vi "Write Send Functionality.vi"(6 "Message Priority":T1=enum."Normal", 7 "Publish Data?(T)":bool=TRUE, 8 "error in (no error)":errorcluster, 9 "Timeout if Waiting(-1ms)":i32=-1, 10 "Send Function(Await Reply)":T2=enum."Await Reply", 11 "Instrument Handler Reponse Msg in":refnum<class "Instrument Handler Response Msg.lvclass">) -> (0 "error out":errorcluster, 3 "Instrument Handler Reponse Msg out":refnum<class "Instrument Handler Response Msg.lvclass">)   [LabVIEW 2020, in "Instrument Handler.lvlib" / "Instrument Handler Response Msg.lvclass"]
doc: "Define the send functionality of the Instrument Handler Reponse Msg."
uses:
  Instrument Handler Response Msg.lvclass
  PPL/HDH.Actor Framework.Core.Publisher.lvlibp/Messages/Response Msg/Response Core/Controls/Ctl_SendFunction.ctl
  PPL/HDH.Actor Framework.Core.Actor.lvlibp/1abvi3w/vi.lib/ActorFramework/Message Enqueuer/Message Priority.ctl
  Instrument Handler Response Msg.lvclass/Instrument Handler Response Msg.ctl
  PPL/HDH.Actor Framework.Core.Publisher.lvlibp
  PPL/HDH.Actor Framework.Core.Actor.lvlibp/1abvi3w/vi.lib/ActorFramework/Message Enqueuer/Message Enqueuer.lvclass
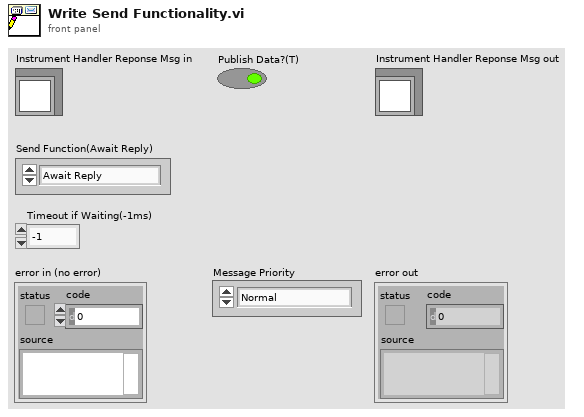
[diagram p1: front panel]
types:
  T1 = typedef "HDH.Actor Framework.Core.Actor.lvlibp/Message Enqueuer.lvclass/Message Priority.ctl" = enum16{"Low", "Normal", "High"}
  T2 = typedef "HDH.Actor Framework.Core.Publisher.lvlibp/Ctl_SendFunction.ctl" = enum16{"Send and Forget", "Request Reply", "Await Reply"}
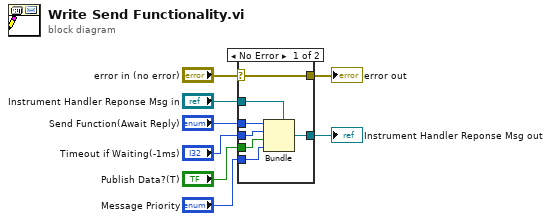
[diagram p0: block diagram]
diagram:
  n1 = case shown="No Error" "error in (no error)" {
    selector: "error in (no error)" -> [w15 w16]
    tunnel: [w15 w16] -> w7
    tunnel: [w13 w17] -> w5
    tunnel: "Instrument Handler Reponse Msg in" -> [w14 w17]
    tunnel: "Send Function(Await Reply)" -> [w12 _]
    tunnel: "Publish Data?(T)" -> [w11 _]
    tunnel: "Timeout if Waiting(-1ms)" -> [w10 _]
    tunnel: "Message Priority" -> [w9 _]
    frame No Error {
      n2 = Bundle(cluster=w14, w12, w10, w11, w9) -> (w13:refnum<class "Instrument Handler Response Msg.lvclass">)
    }
    frame Error {
    }
  }
  "error out" <- w7
  "Instrument Handler Reponse Msg out" <- w5
